vi "PathPlanner_Constraints_FromJSON.vi"(8 "MaxAngularAccRadPSecSq":dbl, 9 "MaxAngularVelRadPsEc;":dbl, 10 "MaxAccelerationMpsSq;":dbl, 11 "MaxVelocityMps;":dbl) -> (3 "PathPlannerConstraints":T1)   [LabVIEW 2019, in "PathPlanner24.lvlib"]
doc: "/**\n * Create a path constraints object from json\n *\n * @param constraintsJson {@link org.json.simple.JSONObject} representing a path constraints\n * object\n * @return The path constraints defined by the given json\n */"
uses:
  PathPlanner24.lvlib
  PathPlannerConstraints.ctl
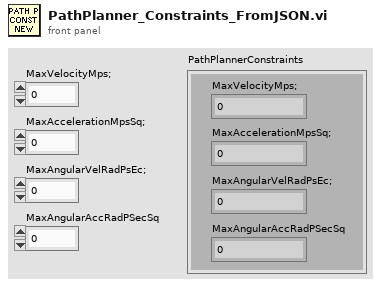
[diagram p1: front panel]
types:
  T1 = typedef "PathPlanner24.lvlib/PathPlannerConstraints.ctl" = cluster{"MaxVelocityMps;":dbl, "MaxAccelerationMpsSq;":dbl, "MaxAngularVelRadPsEc;":dbl, "MaxAngularAccRadPSecSq":dbl}
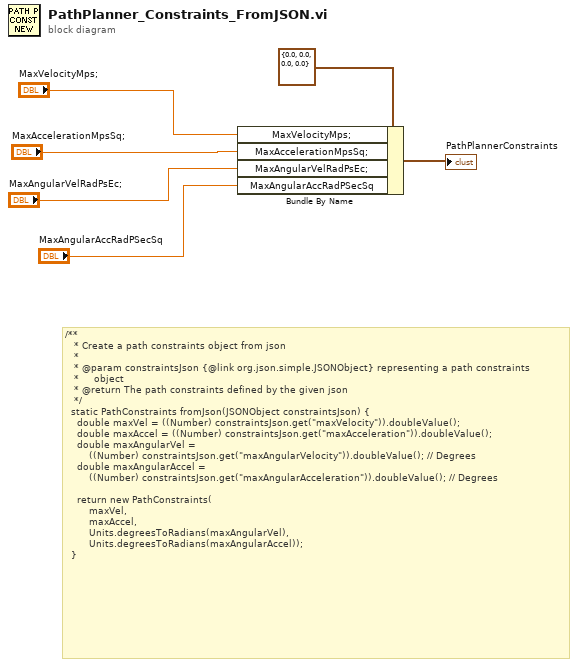
[diagram p0: block diagram]
diagram:
  # "/**\n   * Create a path constraints object from json\n   *\n   * @param constraintsJson {@link org.json.simple.JSONObject} representing a path constraints\n   *     object\n   * @return The path constraints defined by the given json\n   */\n  static PathConstraints fromJson(JSONObject constraintsJson) {\n    double maxVel = ((Number) constraintsJson.get(\"maxVelocity\")).doubleValue();\n    double maxAccel = ((Number) constraintsJson.get(\"maxAcceleration\")).doubleValue();\n    double maxAngularVel =\n        ((Number) constraintsJson.get(\"maxAngularVelocity\")).doubleValue(); // Degrees\n    double maxAngularAccel =\n        ((Number) constraintsJson.get(\"maxAngularAcceleration\")).doubleValue(); // Degrees\n\n    return new PathConstraints(\n        maxVel,\n        maxAccel,\n        Units.degreesToRadians(maxAngularVel),\n        Units.degreesToRadians(maxAngularAccel));\n  }"
  n1 = Bundle By Name(cluster=T1 {"MaxVelocityMps;"=0.0, "MaxAccelerationMpsSq;"=0.0, "MaxAngularVelRadPsEc;"=0.0, "MaxAngularAccRadPSecSq"=0.0} ("PathPlannerConstraints"), "MaxVelocityMps;"="MaxVelocityMps;", "MaxAccelerationMpsSq;"="MaxAccelerationMpsSq;", "MaxAngularVelRadPsEc;"="MaxAngularVelRadPsEc;", "MaxAngularAccRadPSecSq"="MaxAngularAccRadPSecSq") -> (→"PathPlannerConstraints":T1)
